vi "LoopScript_Depinning_External.vi"() -> ()   [LabVIEW 2017]
uses:
  CircleControls.ctl
  ImageAcquisitionProgram/ImageAcquisitionLibrary/GlobalFrontPanelReferences.vi
  AODControl/AODGlobals.vi
  AODControl/MessageQueue/QueueOperations/Enqueue Message (Single).vi
  ImageAcquisitionProgram/ImageAcquisitionLibrary/ImageAcquisitionLibrary.lvlib
  AODControl/AODControl.lvlib
  AODControl/MessageQueue/MessageQueue.lvlib
panel:
  out "Run Number":i32
  out "packing":dbl
  in  "No. of Particles":i32=33
  in  "Run":bool
  in  "Rest Time":dbl=60.0
  in  "No. of Points":i32=33
  out "Total Running \nTime":dbl=90000.0 format="%<%H:%M:%S>t"
  in  "Runs":i32=1
  out "w":dbl[](array[numeric])=[1.0, 1.25, 1.5, 1.75, 2.0]
  in  "w_0":dbl=1.0
  in  "w_f":dbl=2.0
  in  "Steps":i32=5
  in  "R_0":dbl=5.6
  in  "Time":dbl=3600.0
  # "Angular Velocity"
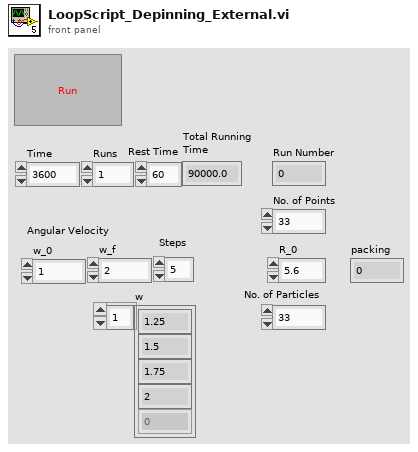
[diagram p1: front panel]
types:
  T1 = typedef "CircleControls.ctl" = cluster{"Radius":dbl, "No. of Points":i32, "Center":cluster{"X":dbl, "Y":dbl}, "Circle":bool, "Density":dbl, "PointSpec":enum32{"No. Of Points", "Density"}, "Hold":bool, "Size":i32, "LatC":dbl, "Eccentricity":dbl, "Phase":dbl}
  T2 = typedef "AODControl.lvlib/MessageQueue.lvlib/All Message Queues.ctl" = cluster{" AOD Interface":refnum<queue>}
  T3 = typedef "ImageAcquisitionLibrary.lvlib/References.ctl" = cluster{"Acquire":refnum<vi>, "Rec":refnum<vi>, "Tracking":refnum<vi>, "Settings":refnum<vi>, "Stop":refnum<vi>, "Initialized?":bool, "ImDisplay":refnum<vi>}
  T4 = typedef "AODControl.lvlib/InterfaceReferences.ctl" = cluster{"AOD Points Display":refnum<vi>, "AOD Array":refnum<vi>, "AOD Array Size":refnum<vi>, "Replace Array List":refnum<vi>, "Replace List":refnum<vi>, "Remove":refnum<vi>, "Index":refnum<vi>, "Move":refnum<vi>, "X":refnum<vi>, "Y":refnum<vi>, "Add":refnum<vi>, "Load":refnum<vi>, "Save":refnum<vi>, "Exit":refnum<vi>, "Dynamic":refnum<vi>, "Rotate":refnum<vi>, "Rotation Speed":refnum<vi>, "Scaling Speed":refnum<vi>, "X Trans Speed":refnum<vi>, "Y Trans Speed":refnum<vi>, "Movie Array":refnum<vi>, "Play":refnum<vi>, "Playing Time":refnum<vi>}
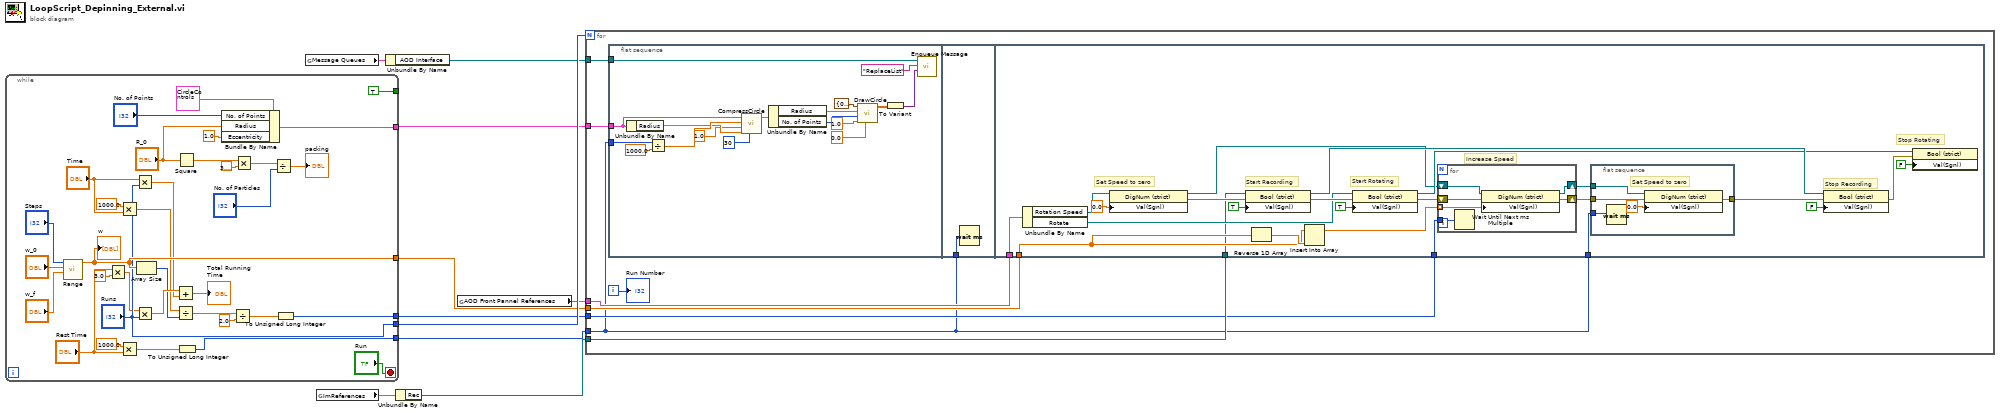
[diagram p0: block diagram]
diagram:
  n1 = while {
    tunnel: [w40] -> w2
    tunnel: [w31] -> w7
    tunnel: [w15] -> w3
    tunnel: [TRUE ("Value (Signaling)")] -> _
    tunnel: ["Runs"] -> w8
    tunnel: [w27] -> w5
    stop <- "Run" stop-if-true
    n2 = call "Range.vi"("End"="w_f", "Start"="w_0", "Steps"="Steps") -> ("Array"=w31:dbl[])  [unwired: 8 in]
    "w" <- w31
    n3 = Multiply(x="Rest Time", y=3.0) -> (x*y=w13:dbl)
    n4 = Multiply(x=1000.0, y="Time") -> (x*y=w18:dbl)
    n5 = Multiply(x=1000.0, y="Rest Time") -> (x*y=w16:dbl)
    n6 = Multiply(x="Time", y="Runs") -> (x*y=w22:dbl)
    n7 = Multiply(x=w13, y="Runs") -> (x*y=w37:dbl)
    n8 = Array Size(array=w31) -> (size(s)=w23:i32)
    n9 = Add(x=w37, y=w22) -> (x+y=→"Total Running \nTime":dbl)
    n10 = Divide(x=w18, y=w23) -> (x/y=w26:dbl)
    n11 = Square(x="R_0") -> (x^2=w43:dbl)
    n12 = To Unsigned Long Integer(number=w16) -> (unsigned 32bit integer=w15:u32)
    n13 = Bundle By Name(cluster=T1 {"Radius"=5.2, "No. of Points"=33, "Center"={"X"=0.0, "Y"=0.0}, "Circle"=TRUE, "Density"=1.0100217542370282, "PointSpec"=enum."No. Of Points", "Hold"=FALSE, "Size"=1, "LatC"=10.0, "Eccentricity"=1.0, "Phase"=0.0} ("Cluster"), "No. of Points"="No. of Points", "Radius"="R_0", "Eccentricity"=1.0) -> (w40:T1)
    n14 = Divide(x=w26, y=2.0) -> (x/y=w24:dbl)
    n15 = Multiply(x=w43, y=3.141592653589793) -> (x*y=w34:dbl)
    n16 = Divide(x=w34, y="No. of Particles") -> (x/y=→"packing":dbl)
    n17 = To Unsigned Long Integer(number=w24) -> (unsigned 32bit integer=w27:u32)
  }
  n18 = global read "AODGlobals.vi" "Message Queues"() -> (w9:T2)
  n19 = global read "GlobalFrontPanelReferences.vi" "ImReferences"() -> (w10:T3)
  n20 = Unbundle By Name(w9) -> ("AOD Interface"=w1:refnum<queue>)
  n21 = Unbundle By Name(w10) -> ("Rec"=w6:refnum<vi>)
  n22 = global read "AODGlobals.vi" "AOD Front Pannel References"() -> (w4:T4)
  n23 = for {
    N: w8 -> [_]
    tunnel: w3 -> [w45]
    tunnel: w7 -> [w51]
    tunnel: w6 -> [w50]
    tunnel: w5 -> [w49]
    tunnel: w4 -> [w48]
    tunnel: w2 -> [w47]
    tunnel: w1 -> [w46]
    i -> [w52]
    n24 = flat-sequence {
      tunnel: w45 -> [w61]
      tunnel: w47 -> [w58]
      tunnel: w46 -> [w53]
      tunnel: w45 -> [w70]
      tunnel: w51 -> [w80]
      tunnel: w45 -> [w79]
      tunnel: w50 -> [w76]
      tunnel: w49 -> [w72]
      tunnel: w48 -> [w71]
      frame #0 {
        n25 = Unbundle By Name(w58) -> ("Radius"=w68:dbl)
        n26 = Divide(x=w61, y=1000.0) -> (x/y=w69:dbl)
        n27 = call "CompressCircle.vi"("Steps"=u32 30, "R0"=w68, "Delta R"=1.0, "Time"=w69, "input ellipse params"=w58) -> ("output ellipse params"=w67:T1)  [unwired: 5 in, 1 out]
        n28 = Unbundle By Name(w67) -> ("Radius"=w64:dbl, "No. of Points"=w65:i32)
        n29 = call "DrawCircle.vi"("Phase"=0.0, "Eccentricity"=1.0, "No Of Points"=w65, "Radius"=w64, "Center"=cluster{"X":dbl, "Y":dbl} {"X"=0.0, "Y"=0.0}) -> ("Array"=w66:dbl[][])  [unwired: 6 in]
        n30 = To Variant(anything=w66) -> (Variant=w63:variant)
        n31 = call-poly "Enqueue Message.vi"("Message Data"=w63, "Message"="ReplaceList", "Message Queue"=w53) -> ()  [unwired: 7 in, 2 out]
      }
      frame #1 {
        n32 = Wait (ms)(milliseconds to wait=w70) -> ()  [unwired: 1 out]
      }
      frame #2 {
        # "Stop Rotating"
        # "Stop Recording"
        # "Increase Speed"
        # "Start Rotating"
        # "Start Recording"
        # "Set Speed to zero"
        n33 = Unbundle By Name(w71) -> ("Rotation Speed"=w81:refnum<vi>, "Rotate"=w82:refnum<vi>)
        n34 = property class="DigNum (strict)"(reference=w81, "Val(Sgnl)"=0.0 ("Value (Signaling)")) -> (reference out=w83:refnum<vi>, error out=w85:errorcluster)  [unwired: 1 in]
        n35 = property class="Bool (strict)"(reference=w76, error in=w85, "Val(Sgnl)"=TRUE ("Value (Signaling)")) -> (reference out=w90:refnum<vi>, error out=w86:errorcluster)
        n36 = Reverse 1D Array(array=w80) -> (reversed array=w91:dbl[])
        n37 = Insert Into Array(array=w80, new element=w91) -> (w92:dbl[])  [unwired: 1 in]
        n38 = property class="Bool (strict)"(reference=w82, error in=w86, "Val(Sgnl)"=TRUE ("Value (Signaling)")) -> (reference out=w89:refnum<vi>, error out=w84:errorcluster)
        n39 = for {
          tunnel: w92 -> [w104] mode=indexing
          shift-right: [w103] -> w93
          shift-left: w83 -> [w105]
          shift-right: [w102] -> w94
          shift-left: w84 -> [w101]
          tunnel: w72 -> [w100]
          n40 = Wait Until Next ms Multiple(millisecond multiple=w100) -> ()  [unwired: 1 out]
          n41 = property class="DigNum (strict)"(reference=w105, error in=w101, "Val(Sgnl)"=w104) -> (reference out=w103:refnum<vi>, error out=w102:errorcluster)
        }
        n42 = flat-sequence {
          tunnel: [w99] -> w88
          tunnel: w93 -> [w97]
          tunnel: w79 -> [w95]
          tunnel: w94 -> [w96]
          frame #0 {
            # "Set Speed to zero"
            n43 = Wait (ms)(milliseconds to wait=w95) -> ()  [unwired: 1 out]
            n44 = property class="DigNum (strict)"(reference=w97, error in=w96, "Val(Sgnl)"=0.0 ("Value (Signaling)")) -> (error out=w99:errorcluster)  [unwired: 1 out]
          }
        }
        n45 = property class="Bool (strict)"(reference=w90, error in=w88, "Val(Sgnl)"=FALSE ("Value (Signaling)")) -> (error out=w87:errorcluster)  [unwired: 1 out]
        n46 = property class="Bool (strict)"(reference=w89, error in=w87, "Val(Sgnl)"=FALSE ("Value (Signaling)")) -> ()  [unwired: 2 out]
      }
    }
    "Run Number" <- w52
  }
